vi "libssh2_session_block_directions.vi"(8 "error in (no error)":errorcluster, 11 "session":T2) -> (0 "error out":errorcluster, 2 "block direction":T1 items=["Inbound"=1, "Outbound"=2])   [LabVIEW 2013, in "libssh2.lvlib"]
doc: "Set the blocking mode for a session.\n\nWhen any of the libssh2 functions return <B>LIBSSH2_ERROR_EAGAIN</B>, a caller should wait for the socket to have data available for reading or writing before calling the function again."
uses:
  libssh2.lvlib
  Session Refnum.ctl
  libssh2_session_block_direction.ctl
  Global Settings.vi
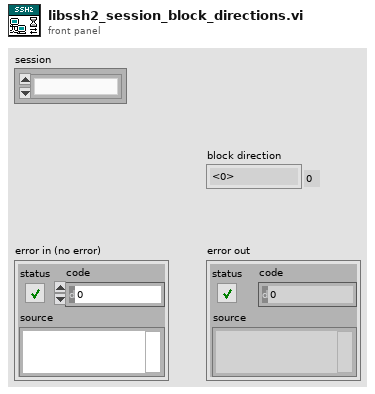
[diagram p1: front panel]
types:
  T1 = typedef "libssh2.lvlib/libssh2_session_block_direction.ctl" = i32
  T2 = typedef "libssh2.lvlib/Session Refnum.ctl" = refnum<k1>
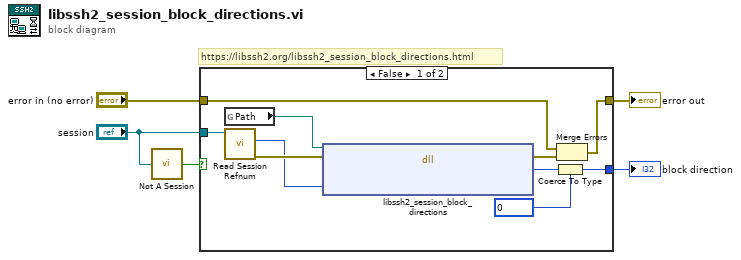
[diagram p0: block diagram]
diagram:
  # "https://libssh2.org/libssh2_session_block_directions.html"
  n1 = call "Not A Session.vi"("session"="session") -> ("Not a Session?"=w1:bool)
  n2 = case shown="False" w1 {
    tunnel: [w11 w16] -> w5
    tunnel: [w7 _] -> w4
    tunnel: "error in (no error)" -> [w12 w16]
    tunnel: "session" -> [w14 _]
    frame False {
      w6 = T1 0 items=["Inbound"=1, "Outbound"=2] ("Ring")
      n3 = global read "Global Settings.vi" "Path"() -> (w9:path)
      n4 = call "Read Session Refnum.vi"("session"=w14) -> ("error out"=w15:errorcluster, "LIBSSH2_SESSION*"=w13:u64)  [unwired: 6 in, 3 out]
      n5 = dll-call lib="?" fn="libssh2_session_block_directions"(path in=w9, error in=w15, "session"=w13) -> (error out=w10:errorcluster, "return value"=w8:i32)  [unwired: 2 in, 1 out]
      n6 = Coerce To Type(0:w8, 1:w6) -> (2:w7:T1)
      n7 = Merge Errors(w12, w10) -> (w11:errorcluster)
    }
    frame True {
    }
  }
  "error out" <- w5
  "block direction" <- w4
